vi "modulator.vi"(1 "C2NI6071E":T9 {"63 ACH63 b100 Libre ?" format="%.3f"; "62 ACH62 b98 Libre ?" format="%.3f"; "61 ACH61 b96 Libre ?" format="%.3f"; "60 ACH60 b94 Libre ?" format="%.3f"; "59 ACH59 b92 Libre ?" format="%.3f"; "58 ACH58 b90 Libre ?" format="%.3f"; "57 ACH57 b88 Libre ?" format="%.3f"; "56 ACH56 b86 Signal laser 1" format="%.3f"; "55 ACH55 b99 Libre ?" format="%.3f"; "54 ACH54 b97 Libre ?" format="%.3f"; "53 ACH53 b95 Libre ?" format="%.3f"; "52 ACH52 b93 Libre ?" format="%.3f"; "51 ACH51 b91 Libre ?" format="%.3f"; "50 ACH50 b89 Libre ?" format="%.3f"; "49 ACH49 b87 Signal laser 2" format="%.3f"; "48 ACH48 b85 Mes position Miroir Y" format="%.3f"; "47 ACH47 b84 Mes position Miroir X" format="%.3f"; "46 ACH46 b82 Mes I obcs Faraday 3" format="%.3f"; "45 ACH45 b80 Mes I obcs Faraday 1" format="%.3f"; "44 ACH44 b78 Mes position Ecran 2" format="%.3f"; "43 ACH43 b74 Mes Fente V position mors B" format="%.3f"; "42 ACH42 b72 Mes Fente H position mors G" format="%.3f"; "41 ACH41 b70 Mes WCM 5" format="%.3f"; "40 ACH40 b68 Mes WCM 3" format="%.3f"; "39 ACH39 b83 Libre ?" format="%.3f"; "38 ACH38 b81 Mes I obcs Faraday 2" format="%.3f"; "37 ACH37 b79 Mes position Ecran 3" format="%.3f"; "36 ACH36 b77 Mes position Ecran 1" format="%.3f"; "35 ACH35 b73 Mes Fente V position mors H" format="%.3f"; "34 ACH34 b71 Mes Fente H position mors D" format="%.3f"; "33 ACH33 b69 Mes WCM 4" format="%.3f"; "32 ACH32 b67 Mes WCM 2D" format="%.3f"; "31 ACH31 b66 Mes WCM 2G" format="%.3f"; "30 ACH30 b64 Mes WCM 2H" format="%.3f"; "29 ACH29 b62 Mes WCM 1G" format="%.3f"; "28 ACH28 b60 Mes WCM 1H" format="%.3f"; "27 ACH27 b58 Mes I Faraday 2" format="%.3f"; "26 ACH26 b56 Mes HF directe Section" format="%.3f"; "25 ACH25 b54 Réservé" format="%.3f"; "24 ACH24 b52 Mes I Klystron" format="%.3f"; "23 ACH23 b65 Mes WCM 2B" format="%.3f"; "22 ACH22 b63 Mes WCM 1D" format="%.3f"; "21 ACH21 b61 Mes WCM 1B" format="%.3f"; "20 ACH20 b59 Mes I Faraday 3" format="%.3f"; "19 ACH19 b57 Mes I Faraday 1" format="%.3f"; "18 ACH18 b55 Mes HF directe Canon" format="%.3f"; "17 ACH17 b53 Mes V LAR" format="%.3f"; "16 ACH16 b51 Mes V Klystron" format="%.3f"; "15 ACH15 b18 Mes I alimentation HT" format="%.3f"; "14 ACH14 b16 Libre ?" format="%.3f"; "13 ACH13 b14 Mes I Focalisateur 2" format="%.3f"; "12 ACH12 b12 Mes I fin de Ligne" format="%.3f"; "11 ACH11 b10 Mes I Thyratron" format="%.3f"; "10 ACH10 b08 Mes I Réservoir Thyratron" format="%.3f"; "09 ACH09 b06 Mes I  Chauffage Klystron" format="%.3f"; "08 ACH08 b04 Mes I Chauffage Thyratron" format="%.3f"; "07 ACH07 b17 Mes V alimentation HT" format="%.3f"; "06 ACH06 b15 Mes I Focalisateur 3" format="%.3f"; "05 ACH05 b13 Mes I Focalisateur 1" format="%.3f"; "04 ACH04 b11 Mes I Prémagnétisation" format="%.3f"; "03 ACH03 b09 Réservé" format="%.3f"; "02 ACH02 b07 Mes I D'Qing" format="%.3f"; "01 ACH01 b05 Mes V Chauffage Klystron" format="%.3f"; "00 ACH00 b03 Mes V Chauffage Thyratron" format="%.3f"}, 2 "archive in":T1={"sync"={"elyse/sync/NI6071E/delay"=1.5500000000000005, "elyse/sync/NI6071E/width"=1.0, "elyse/sync/frequency/delay"=10.0, "elyse/sync/frequency/width"=181000.0, "elyse/sync/WCM/delay"=2177.9, "elyse/sync/WCM/width"=10.0, "elyse/sync/modulator/delay"=2182.400000000002, "elyse/sync/modulator/width"=3.0, "elyse/sync/HF/delay"=2175.0, "elyse/sync/HF/width"=3.0, "elyse/sync/Faraday/delay"=5080.0, "elyse/sync/Faraday/width"=100.0, "elyse/sync/Oscilloscope/delay"=2175.0, "elyse/sync/Oscilloscope/width"=2.8, "elyse/sync/50Hz_20MHz/delay"=1.0, "elyse/sync/50Hz_20MHz/width"=5000.0, "elyse/sync/laser_HF/delay"=0.35, "elyse/sync/laser_HF/width"=0.35, "elyse/sync/IMAC/delay"=2176.0, "elyse/sync/IMAC/width"=100.0, "elyse/sync/laser/delay"=2008.3, "elyse/sync/laser/width"=10.0, "elyse/sync/oscilloscope1/delay"=2175.0, "elyse/sync/oscilloscope1/width"=10.0, "elyse/sync/oscilloscope2/delay"=2175.0, "elyse/sync/oscilloscope2/width"=100.0, "elyse/sync/detection1/delay"=500.0, "elyse/sync/detection1/width"=500.0, "elyse/sync/detection1/delay"=0.3, "elyse/sync/detection2/width"=10.0, "elyse/sync/machine/delay"=2175.0, "elyse/sync/machine/width"=100.0, "elyse/sync/n_selection"=4.0}, "HT"={"elyse/HT/voltage/set_value"=6.5, "elyse/HT/voltage/value"=1.5625e-08, "elyse/HT/current/value"=0.0, "elyse/preamplifier/set_value"=1.5625e-08, "elyse/preamplifier/value"=0.0}, "HF"={"elyse/HF/attenuator/value"=-0.01903046052094623, "elyse/HF/dephaser/value"=-18.585806237727724, "elyse/HF/dephaser/value_manuel"=-78.82860725035081, "elyse/HF/canon/value"=0.0, "elyse/HF/section/value"=-18.585806237727724}, "vacuum"={"elyse/vacuum/preparation_chamber/state"=TRUE, "elyse/vacuum/preparation_chamber/measurement"=0.0, "elyse/vacuum/HF/state"=TRUE, "elyse/vacuum/HF/measurement"=0.0, "elyse/vacuum/canon/state"=TRUE, "elyse/vacuum/canon/measurement"=0.0, "elyse/vacuum/section/state"=TRUE, "elyse/vacuum/section/measurement"=0.0, "elyse/vacuum/dipole1/state"=TRUE, "elyse/vacuum/dipole1/measurement"=0.0, "elyse/vacuum/screen1/state"=TRUE, "elyse/vacuum/screen1/measurement"=0.0, "elyse/vacuum/mirror/state"=TRUE, "elyse/vacuum/mirror/measurement"=0.0, "elyse/vacuum/tpg300_section/state"=TRUE, "elyse/vacuum/tpg300_section/measurement"=0.0, "elyse/vacuum/valves/cathode/state"=FALSE, "elyse/vacuum/valves/injection/state"=FALSE}, "modulator"={"elyse/modulator/focale1/current/value"=0.0, "elyse/modulator/focale2/current/value"=0.0, "elyse/modulator/focale3/current/value"=0.0, "elyse/modulator/LAR/voltage/value"=0.0, "elyse/modulator/line_end/current/value"=0.0, "elyse/modulator/thyratron/currents/power/value"=0.0, "elyse/modulator/thyratron_reservoir/current/value"=0.0, "elyse/modulator/paramagnetization/current/value"=0.0, "elyse/modulator/thyratron/voltages/heating/value"=0.0, "elyse/modulator/thyratron/currents/heating/value"=0.0, "elyse/modulator/klystron/currents/power/value"=0.0, "elyse/modulator/klystron/voltages/power/value"=0.0, "elyse/modulator/klystron/currents/heating/value"=0.0, "elyse/modulator/klystron/voltages/heating/value"=0.0}, "cooling"={"elyse/cooling/section/temperature/set_value"=28.0, "elyse/cooling/section/temperature/measurement"=27.96142578125, "elyse/cooling/canon/temperature/set_value"=20.2, "elyse/cooling/canon/temperature/measurement"=26.69921875}, "magnets"={"elyse/magnets/focale/set_value"=0.0, "elyse/magnets/focale/value"=0.0, "elyse/magnets/phase_HF_laser/set_value"=0.0, "elyse/magnets/phase_HF_laser/value"=0.0, "elyse/magnets/dipole1/set_value"=0.0, "elyse/magnets/dipole1/value"=0.0, "elyse/magnets/dipole2/set_value"=0.0, "elyse/magnets/dipole2/value"=0.0, "elyse/magnets/Cor_H1/set_value"=0.0, "elyse/magnets/Cor_H1/value"=0.0, "elyse/magnets/Cor_V1/set_value"=0.0, "elyse/magnets/Cor_V1/value"=0.0, "elyse/magnets/Cor_H2/set_value"=0.0, "elyse/magnets/Cor_H2/value"=0.0, "elyse/magnets/Cor_V2/set_value"=0.0, "elyse/magnets/Cor_V2/value"=0.0, "elyse/magnets/Cor_H3/set_value"=0.0, "elyse/magnets/Cor_H3/value"=0.0, "elyse/magnets/Cor_V3/set_value"=-5.0, "elyse/magnets/Cor_V3/value"=0.0, "elyse/magnets/Cor_H4/set_value"=0.0, "elyse/magnets/Cor_H4/value"=0.0, "elyse/magnets/Cor_V4/set_value"=0.0, "elyse/magnets/Cor_V4/value"=0.0, "elyse/magnets/Cor_H5/set_value"=0.0, "elyse/magnets/Cor_H5/value"=0.0, "elyse/magnets/Cor_V5/set_value"=0.0, "elyse/magnets/Cor_V5/value"=0.0, "elyse/magnets/triplet1-1/set_value"=0.0, "elyse/magnets/triplet1-1/value"=0.0, "elyse/magnets/triplet1-2/set_value"=0.0, "elyse/magnets/triplet1-2/value"=0.0, "elyse/magnets/triplet2-1/set_value"=0.0, "elyse/magnets/triplet2-1/value"=0.0, "elyse/magnets/triplet2-2/set_value"=0.0, "elyse/magnets/triplet2-2/value"=0.0, "elyse/magnets/qudrupole1/set_value"=0.0, "elyse/magnets/qudrupole1/value"=0.0, "elyse/magnets/qudrupole2/set_value"=0.0, "elyse/magnets/qudrupole2/value"=0.0}, "time"={"elyse/timestamp"=0.0}}) -> (0 "archive out":T1={"sync"={"elyse/sync/NI6071E/delay"=1.5500000000000005, "elyse/sync/NI6071E/width"=1.0, "elyse/sync/frequency/delay"=10.0, "elyse/sync/frequency/width"=181000.0, "elyse/sync/WCM/delay"=2177.9, "elyse/sync/WCM/width"=10.0, "elyse/sync/modulator/delay"=2182.400000000002, "elyse/sync/modulator/width"=3.0, "elyse/sync/HF/delay"=2175.0, "elyse/sync/HF/width"=3.0, "elyse/sync/Faraday/delay"=5080.0, "elyse/sync/Faraday/width"=100.0, "elyse/sync/Oscilloscope/delay"=2175.0, "elyse/sync/Oscilloscope/width"=2.8, "elyse/sync/50Hz_20MHz/delay"=1.0, "elyse/sync/50Hz_20MHz/width"=5000.0, "elyse/sync/laser_HF/delay"=0.35, "elyse/sync/laser_HF/width"=0.35, "elyse/sync/IMAC/delay"=2176.0, "elyse/sync/IMAC/width"=100.0, "elyse/sync/laser/delay"=2008.3, "elyse/sync/laser/width"=10.0, "elyse/sync/oscilloscope1/delay"=2175.0, "elyse/sync/oscilloscope1/width"=10.0, "elyse/sync/oscilloscope2/delay"=2175.0, "elyse/sync/oscilloscope2/width"=100.0, "elyse/sync/detection1/delay"=500.0, "elyse/sync/detection1/width"=500.0, "elyse/sync/detection1/delay"=0.3, "elyse/sync/detection2/width"=10.0, "elyse/sync/machine/delay"=2175.0, "elyse/sync/machine/width"=100.0, "elyse/sync/n_selection"=4.0}, "HT"={"elyse/HT/voltage/set_value"=6.5, "elyse/HT/voltage/value"=1.5625e-08, "elyse/HT/current/value"=0.0, "elyse/preamplifier/set_value"=1.5625e-08, "elyse/preamplifier/value"=0.0}, "HF"={"elyse/HF/attenuator/value"=-0.01903046052094623, "elyse/HF/dephaser/value"=-18.585806237727724, "elyse/HF/dephaser/value_manuel"=-78.82860725035081, "elyse/HF/canon/value"=0.0, "elyse/HF/section/value"=-18.585806237727724}, "vacuum"={"elyse/vacuum/preparation_chamber/state"=TRUE, "elyse/vacuum/preparation_chamber/measurement"=0.0, "elyse/vacuum/HF/state"=TRUE, "elyse/vacuum/HF/measurement"=0.0, "elyse/vacuum/canon/state"=TRUE, "elyse/vacuum/canon/measurement"=0.0, "elyse/vacuum/section/state"=TRUE, "elyse/vacuum/section/measurement"=0.0, "elyse/vacuum/dipole1/state"=TRUE, "elyse/vacuum/dipole1/measurement"=0.0, "elyse/vacuum/screen1/state"=TRUE, "elyse/vacuum/screen1/measurement"=0.0, "elyse/vacuum/mirror/state"=TRUE, "elyse/vacuum/mirror/measurement"=0.0, "elyse/vacuum/tpg300_section/state"=TRUE, "elyse/vacuum/tpg300_section/measurement"=0.0, "elyse/vacuum/valves/cathode/state"=FALSE, "elyse/vacuum/valves/injection/state"=FALSE}, "modulator"={"elyse/modulator/focale1/current/value"=0.0, "elyse/modulator/focale2/current/value"=0.0, "elyse/modulator/focale3/current/value"=0.0, "elyse/modulator/LAR/voltage/value"=0.0, "elyse/modulator/line_end/current/value"=0.0, "elyse/modulator/thyratron/currents/power/value"=0.0, "elyse/modulator/thyratron_reservoir/current/value"=0.0, "elyse/modulator/paramagnetization/current/value"=0.0, "elyse/modulator/thyratron/voltages/heating/value"=0.0, "elyse/modulator/thyratron/currents/heating/value"=0.0, "elyse/modulator/klystron/currents/power/value"=0.0, "elyse/modulator/klystron/voltages/power/value"=0.0, "elyse/modulator/klystron/currents/heating/value"=0.0, "elyse/modulator/klystron/voltages/heating/value"=0.0}, "cooling"={"elyse/cooling/section/temperature/set_value"=28.0, "elyse/cooling/section/temperature/measurement"=27.96142578125, "elyse/cooling/canon/temperature/set_value"=20.2, "elyse/cooling/canon/temperature/measurement"=26.69921875}, "magnets"={"elyse/magnets/focale/set_value"=0.0, "elyse/magnets/focale/value"=0.0, "elyse/magnets/phase_HF_laser/set_value"=0.0, "elyse/magnets/phase_HF_laser/value"=0.0, "elyse/magnets/dipole1/set_value"=0.0, "elyse/magnets/dipole1/value"=0.0, "elyse/magnets/dipole2/set_value"=0.0, "elyse/magnets/dipole2/value"=0.0, "elyse/magnets/Cor_H1/set_value"=0.0, "elyse/magnets/Cor_H1/value"=0.0, "elyse/magnets/Cor_V1/set_value"=0.0, "elyse/magnets/Cor_V1/value"=0.0, "elyse/magnets/Cor_H2/set_value"=0.0, "elyse/magnets/Cor_H2/value"=0.0, "elyse/magnets/Cor_V2/set_value"=0.0, "elyse/magnets/Cor_V2/value"=0.0, "elyse/magnets/Cor_H3/set_value"=0.0, "elyse/magnets/Cor_H3/value"=0.0, "elyse/magnets/Cor_V3/set_value"=-5.0, "elyse/magnets/Cor_V3/value"=0.0, "elyse/magnets/Cor_H4/set_value"=0.0, "elyse/magnets/Cor_H4/value"=0.0, "elyse/magnets/Cor_V4/set_value"=0.0, "elyse/magnets/Cor_V4/value"=0.0, "elyse/magnets/Cor_H5/set_value"=0.0, "elyse/magnets/Cor_H5/value"=0.0, "elyse/magnets/Cor_V5/set_value"=0.0, "elyse/magnets/Cor_V5/value"=0.0, "elyse/magnets/triplet1-1/set_value"=0.0, "elyse/magnets/triplet1-1/value"=0.0, "elyse/magnets/triplet1-2/set_value"=0.0, "elyse/magnets/triplet1-2/value"=0.0, "elyse/magnets/triplet2-1/set_value"=0.0, "elyse/magnets/triplet2-1/value"=0.0, "elyse/magnets/triplet2-2/set_value"=0.0, "elyse/magnets/triplet2-2/value"=0.0, "elyse/magnets/qudrupole1/set_value"=0.0, "elyse/magnets/qudrupole1/value"=0.0, "elyse/magnets/qudrupole2/set_value"=0.0, "elyse/magnets/qudrupole2/value"=0.0}, "time"={"elyse/timestamp"=0.0}})   [LabVIEW 2020]
uses:
  archive.ctl
  sync_type_def.ctl
  HT_type-def.ctl
  HF_type_def.ctl
  vacuum_type_def.ctl
  modulator_type_def.ctl
  water_cooling_type_def.ctl
  all_magnets_type_def.ctl
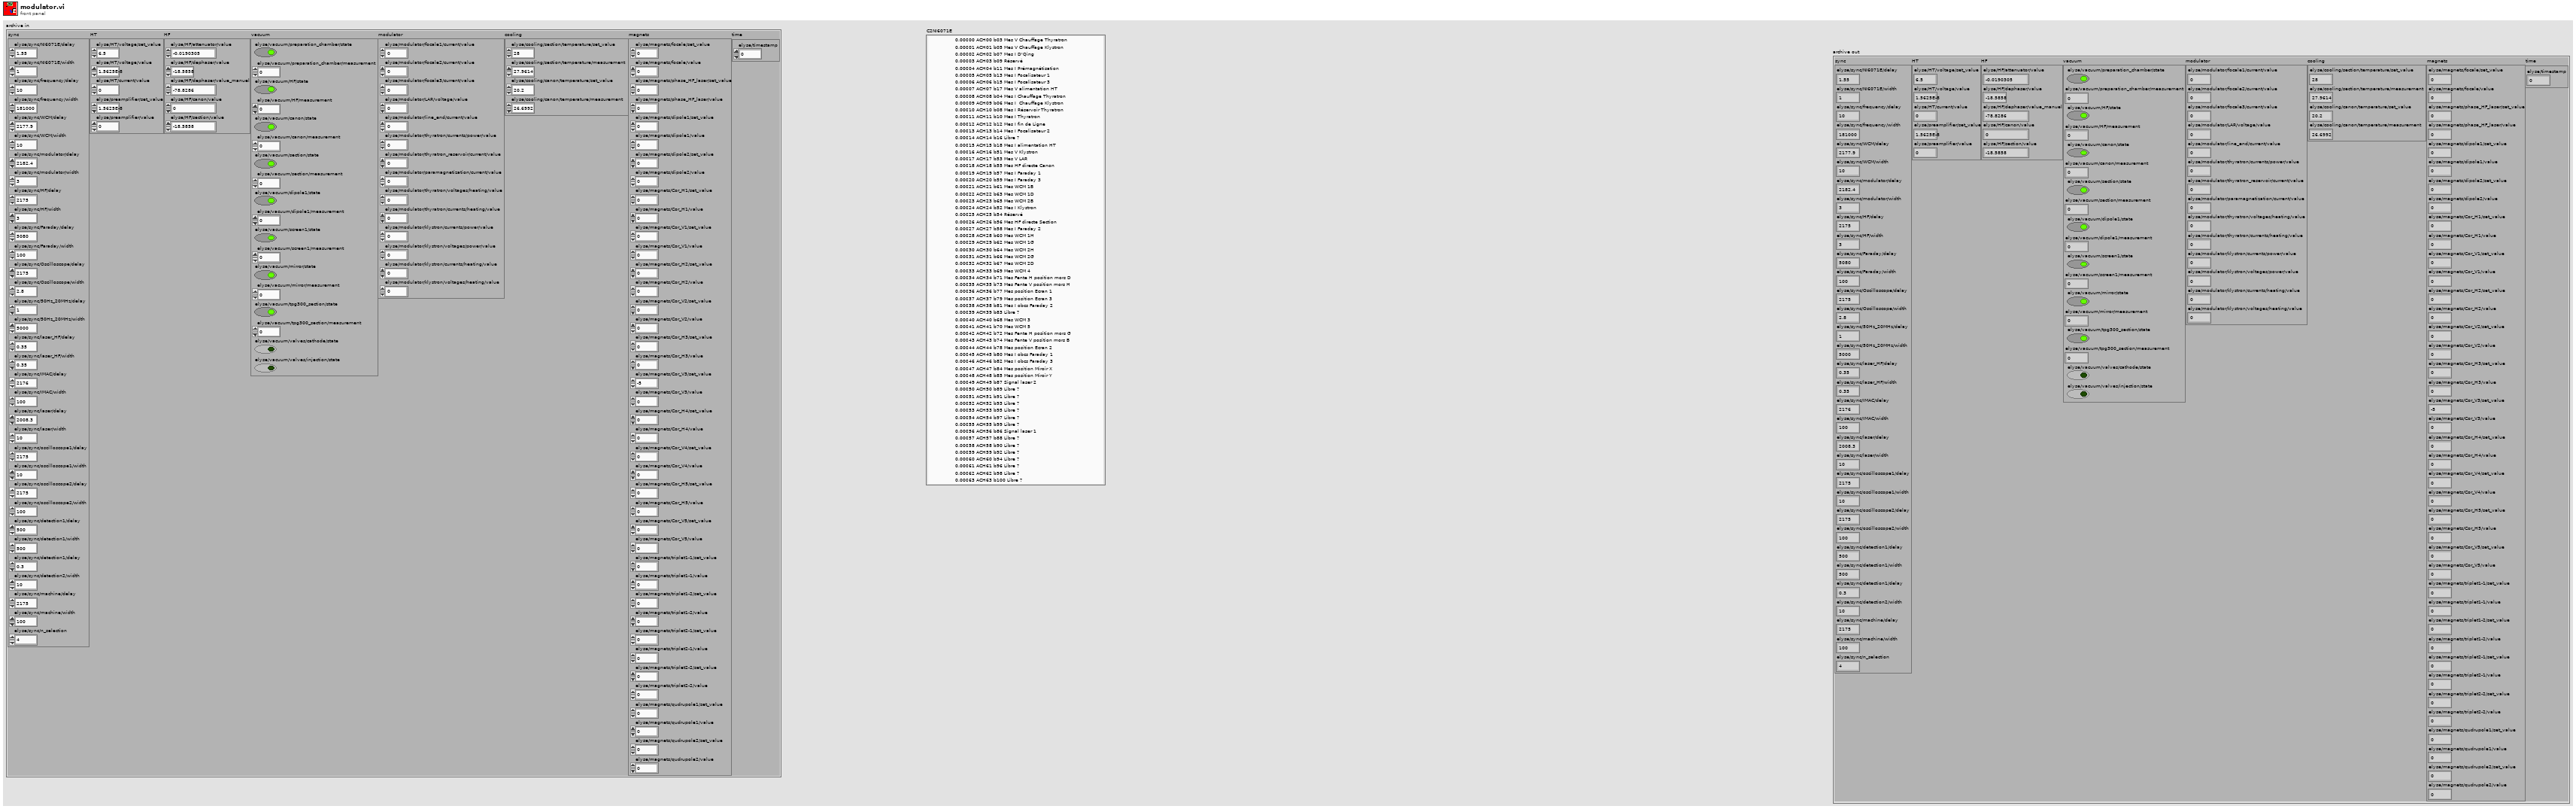
[diagram p1: front panel]
types:
  T1 = typedef "archive.ctl" = cluster{"sync":T2, "HT":T3, "HF":T4, "vacuum":T5, "modulator":T6, "cooling":T7, "magnets":T8, "time":cluster{"elyse/timestamp":dbl}}
  T2 = typedef "sync_type_def.ctl" = cluster{"elyse/sync/NI6071E/delay":dbl, "elyse/sync/NI6071E/width":dbl, "elyse/sync/frequency/delay":dbl, "elyse/sync/frequency/width":dbl, "elyse/sync/WCM/delay":dbl, "elyse/sync/WCM/width":dbl, "elyse/sync/modulator/delay":dbl, "elyse/sync/modulator/width":dbl, "elyse/sync/HF/delay":dbl, "elyse/sync/HF/width":dbl, "elyse/sync/Faraday/delay":dbl, "elyse/sync/Faraday/width":dbl, "elyse/sync/Oscilloscope/delay":dbl, "elyse/sync/Oscilloscope/width":dbl, "elyse/sync/50Hz_20MHz/delay":dbl, "elyse/sync/50Hz_20MHz/width":dbl, "elyse/sync/laser_HF/delay":dbl, "elyse/sync/laser_HF/width":dbl, "elyse/sync/IMAC/delay":dbl, "elyse/sync/IMAC/width":dbl, "elyse/sync/laser/delay":dbl, "elyse/sync/laser/width":dbl, "elyse/sync/oscilloscope1/delay":dbl, "elyse/sync/oscilloscope1/width":dbl, "elyse/sync/oscilloscope2/delay":dbl, "elyse/sync/oscilloscope2/width":dbl, "elyse/sync/detection1/delay":dbl, "elyse/sync/detection1/width":dbl, "elyse/sync/detection1/delay":dbl, "elyse/sync/detection2/width":dbl, "elyse/sync/machine/delay":dbl, "elyse/sync/machine/width":dbl, "elyse/sync/n_selection":dbl}
  T3 = typedef "HT_type-def.ctl" = cluster{"elyse/HT/voltage/set_value":dbl, "elyse/HT/voltage/value":dbl, "elyse/HT/current/value":dbl, "elyse/preamplifier/set_value":dbl, "elyse/preamplifier/value":dbl}
  T4 = typedef "HF_type_def.ctl" = cluster{"elyse/HF/attenuator/value":dbl, "elyse/HF/dephaser/value":dbl, "elyse/HF/dephaser/value_manuel":dbl, "elyse/HF/canon/value":dbl, "elyse/HF/section/value":dbl}
  T5 = typedef "vacuum_type_def.ctl" = cluster{"elyse/vacuum/preparation_chamber/state":bool, "elyse/vacuum/preparation_chamber/measurement":dbl, "elyse/vacuum/HF/state":bool, "elyse/vacuum/HF/measurement":dbl, "elyse/vacuum/canon/state":bool, "elyse/vacuum/canon/measurement":dbl, "elyse/vacuum/section/state":bool, "elyse/vacuum/section/measurement":dbl, "elyse/vacuum/dipole1/state":bool, "elyse/vacuum/dipole1/measurement":dbl, "elyse/vacuum/screen1/state":bool, "elyse/vacuum/screen1/measurement":dbl, "elyse/vacuum/mirror/state":bool, "elyse/vacuum/mirror/measurement":dbl, "elyse/vacuum/tpg300_section/state":bool, "elyse/vacuum/tpg300_section/measurement":dbl, "elyse/vacuum/valves/cathode/state":bool, "elyse/vacuum/valves/injection/state":bool}
  T6 = typedef "modulator_type_def.ctl" = cluster{"elyse/modulator/focale1/current/value":dbl, "elyse/modulator/focale2/current/value":dbl, "elyse/modulator/focale3/current/value":dbl, "elyse/modulator/LAR/voltage/value":dbl, "elyse/modulator/line_end/current/value":dbl, "elyse/modulator/thyratron/currents/power/value":dbl, "elyse/modulator/thyratron_reservoir/current/value":dbl, "elyse/modulator/paramagnetization/current/value":dbl, "elyse/modulator/thyratron/voltages/heating/value":dbl, "elyse/modulator/thyratron/currents/heating/value":dbl, "elyse/modulator/klystron/currents/power/value":dbl, "elyse/modulator/klystron/voltages/power/value":dbl, "elyse/modulator/klystron/currents/heating/value":dbl, "elyse/modulator/klystron/voltages/heating/value":dbl}
  T7 = typedef "water_cooling_type_def.ctl" = cluster{"elyse/cooling/section/temperature/set_value":dbl, "elyse/cooling/section/temperature/measurement":dbl, "elyse/cooling/canon/temperature/set_value":dbl, "elyse/cooling/canon/temperature/measurement":dbl}
  T8 = typedef "all_magnets_type_def.ctl" = cluster{"elyse/magnets/focale/set_value":dbl, "elyse/magnets/focale/value":dbl, "elyse/magnets/phase_HF_laser/set_value":dbl, "elyse/magnets/phase_HF_laser/value":dbl, "elyse/magnets/dipole1/set_value":dbl, "elyse/magnets/dipole1/value":dbl, "elyse/magnets/dipole2/set_value":dbl, "elyse/magnets/dipole2/value":dbl, "elyse/magnets/Cor_H1/set_value":dbl, "elyse/magnets/Cor_H1/value":dbl, "elyse/magnets/Cor_V1/set_value":dbl, "elyse/magnets/Cor_V1/value":dbl, "elyse/magnets/Cor_H2/set_value":dbl, "elyse/magnets/Cor_H2/value":dbl, "elyse/magnets/Cor_V2/set_value":dbl, "elyse/magnets/Cor_V2/value":dbl, "elyse/magnets/Cor_H3/set_value":dbl, "elyse/magnets/Cor_H3/value":dbl, "elyse/magnets/Cor_V3/set_value":dbl, "elyse/magnets/Cor_V3/value":dbl, "elyse/magnets/Cor_H4/set_value":dbl, "elyse/magnets/Cor_H4/value":dbl, "elyse/magnets/Cor_V4/set_value":dbl, "elyse/magnets/Cor_V4/value":dbl, "elyse/magnets/Cor_H5/set_value":dbl, "elyse/magnets/Cor_H5/value":dbl, "elyse/magnets/Cor_V5/set_value":dbl, "elyse/magnets/Cor_V5/value":dbl, "elyse/magnets/triplet1-1/set_value":dbl, "elyse/magnets/triplet1-1/value":dbl, "elyse/magnets/triplet1-2/set_value":dbl, "elyse/magnets/triplet1-2/value":dbl, "elyse/magnets/triplet2-1/set_value":dbl, "elyse/magnets/triplet2-1/value":dbl, "elyse/magnets/triplet2-2/set_value":dbl, "elyse/magnets/triplet2-2/value":dbl, "elyse/magnets/qudrupole1/set_value":dbl, "elyse/magnets/qudrupole1/value":dbl, "elyse/magnets/qudrupole2/set_value":dbl, "elyse/magnets/qudrupole2/value":dbl}
  T9 = cluster{"00 ACH00 b03 Mes V Chauffage Thyratron":dbl, "01 ACH01 b05 Mes V Chauffage Klystron":dbl, "02 ACH02 b07 Mes I D'Qing":dbl, "03 ACH03 b09 Réservé":dbl, "04 ACH04 b11 Mes I Prémagnétisation":dbl, "05 ACH05 b13 Mes I Focalisateur 1":dbl, "06 ACH06 b15 Mes I Focalisateur 3":dbl, "07 ACH07 b17 Mes V alimentation HT":dbl, "08 ACH08 b04 Mes I Chauffage Thyratron":dbl, "09 ACH09 b06 Mes I  Chauffage Klystron":dbl, "10 ACH10 b08 Mes I Réservoir Thyratron":dbl, "11 ACH11 b10 Mes I Thyratron":dbl, "12 ACH12 b12 Mes I fin de Ligne":dbl, "13 ACH13 b14 Mes I Focalisateur 2":dbl, "14 ACH14 b16 Libre ?":dbl, "15 ACH15 b18 Mes I alimentation HT":dbl, "16 ACH16 b51 Mes V Klystron":dbl, "17 ACH17 b53 Mes V LAR":dbl, "18 ACH18 b55 Mes HF directe Canon":dbl, "19 ACH19 b57 Mes I Faraday 1":dbl, "20 ACH20 b59 Mes I Faraday 3":dbl, "21 ACH21 b61 Mes WCM 1B":dbl, "22 ACH22 b63 Mes WCM 1D":dbl, "23 ACH23 b65 Mes WCM 2B":dbl, "24 ACH24 b52 Mes I Klystron":dbl, "25 ACH25 b54 Réservé":dbl, "26 ACH26 b56 Mes HF directe Section":dbl, "27 ACH27 b58 Mes I Faraday 2":dbl, "28 ACH28 b60 Mes WCM 1H":dbl, "29 ACH29 b62 Mes WCM 1G":dbl, "30 ACH30 b64 Mes WCM 2H":dbl, "31 ACH31 b66 Mes WCM 2G":dbl, "32 ACH32 b67 Mes WCM 2D":dbl, "33 ACH33 b69 Mes WCM 4":dbl, "34 ACH34 b71 Mes Fente H position mors D":dbl, "35 ACH35 b73 Mes Fente V position mors H":dbl, "36 ACH36 b77 Mes position Ecran 1":dbl, "37 ACH37 b79 Mes position Ecran 3":dbl, "38 ACH38 b81 Mes I obcs Faraday 2":dbl, "39 ACH39 b83 Libre ?":dbl, "40 ACH40 b68 Mes WCM 3":dbl, "41 ACH41 b70 Mes WCM 5":dbl, "42 ACH42 b72 Mes Fente H position mors G":dbl, "43 ACH43 b74 Mes Fente V position mors B":dbl, "44 ACH44 b78 Mes position Ecran 2":dbl, "45 ACH45 b80 Mes I obcs Faraday 1":dbl, "46 ACH46 b82 Mes I obcs Faraday 3":dbl, "47 ACH47 b84 Mes position Miroir X":dbl, "48 ACH48 b85 Mes position Miroir Y":dbl, "49 ACH49 b87 Signal laser 2":dbl, "50 ACH50 b89 Libre ?":dbl, "51 ACH51 b91 Libre ?":dbl, "52 ACH52 b93 Libre ?":dbl, "53 ACH53 b95 Libre ?":dbl, "54 ACH54 b97 Libre ?":dbl, "55 ACH55 b99 Libre ?":dbl, "56 ACH56 b86 Signal laser 1":dbl, "57 ACH57 b88 Libre ?":dbl, "58 ACH58 b90 Libre ?":dbl, "59 ACH59 b92 Libre ?":dbl, "60 ACH60 b94 Libre ?":dbl, "61 ACH61 b96 Libre ?":dbl, "62 ACH62 b98 Libre ?":dbl, "63 ACH63 b100 Libre ?":dbl}
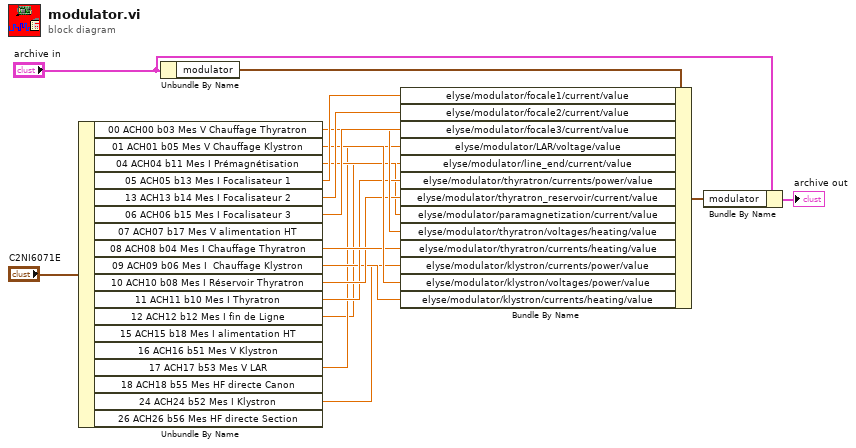
[diagram p0: block diagram]
diagram:
  n1 = Unbundle By Name("C2NI6071E") -> ("00 ACH00 b03 Mes V Chauffage Thyratron"=w10:dbl, "01 ACH01 b05 Mes V Chauffage Klystron"=w9:dbl, "04 ACH04 b11 Mes I Prémagnétisation"=w4:dbl, "05 ACH05 b13 Mes I Focalisateur 1"=w13:dbl, "13 ACH13 b14 Mes I Focalisateur 2"=w12:dbl, "06 ACH06 b15 Mes I Focalisateur 3"=w11:dbl, "08 ACH08 b04 Mes I Chauffage Thyratron"=w8:dbl, "09 ACH09 b06 Mes I  Chauffage Klystron"=w5:dbl, "10 ACH10 b08 Mes I Réservoir Thyratron"=w7:dbl, "11 ACH11 b10 Mes I Thyratron"=w6:dbl, "12 ACH12 b12 Mes I fin de Ligne"=w1:dbl, "17 ACH17 b53 Mes V LAR"=w2:dbl, "24 ACH24 b52 Mes I Klystron"=w3:dbl)  [unwired: 5 out]
  n2 = Unbundle By Name("archive in") -> ("modulator"=w17:T6)
  n3 = Bundle By Name(cluster=w17, "elyse/modulator/focale1/current/value"=w13, "elyse/modulator/focale2/current/value"=w12, "elyse/modulator/focale3/current/value"=w11, "elyse/modulator/LAR/voltage/value"=w2, "elyse/modulator/line_end/current/value"=w1, "elyse/modulator/thyratron/currents/power/value"=w6, "elyse/modulator/thyratron_reservoir/current/value"=w7, "elyse/modulator/paramagnetization/current/value"=w4, "elyse/modulator/thyratron/voltages/heating/value"=w10, "elyse/modulator/thyratron/currents/heating/value"=w8, "elyse/modulator/klystron/currents/power/value"=w3, "elyse/modulator/klystron/voltages/power/value"=w9, "elyse/modulator/klystron/currents/heating/value"=w5) -> (w15:T6)
  n4 = Bundle By Name(cluster="archive in", "modulator"=w15) -> (→"archive out":T1)
